vi "GT Compile.vi"(8 "error in (no error)":errorcluster caption="错误输入（无错误）", 9 "pWrongInfo":T1, 10 "pFileName":string, 11 "cardNum":i16) -> (0 "error out":errorcluster caption="错误输出", 1 "pWrongInfo out":T1, 2 "pFileName out":string, 3 "pFileName":string, 4 "function return":i16, 5 "pMessage":string)   [LabVIEW 2020, in "gts.lvlib"]
doc: "GT_API GT_Compile(short cardNum,char *pFileName,TCompileInfo *pWrongInfo);"
uses:
  gts.lvlib
  <vilib>/Utility/importsl/GetValueByPointer/datatype.ctl
  <vilib>/Utility/importsl/GetValueByPointer/GetValueByPointer.xnode
  dll/32bit/multi_card/gts.dll
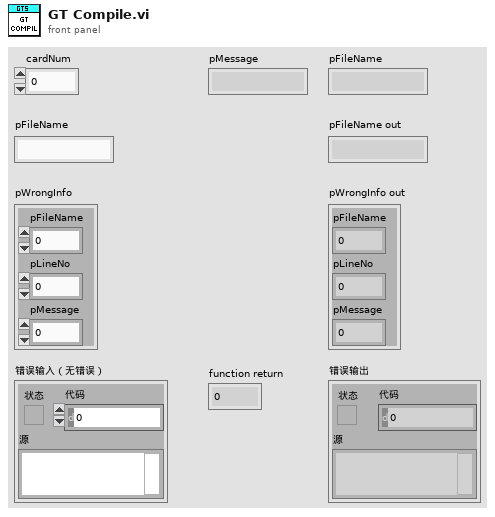
[diagram p1: front panel]
types:
  T1 = cluster{"pFileName":u32, "pLineNo":u32, "pMessage":u32}
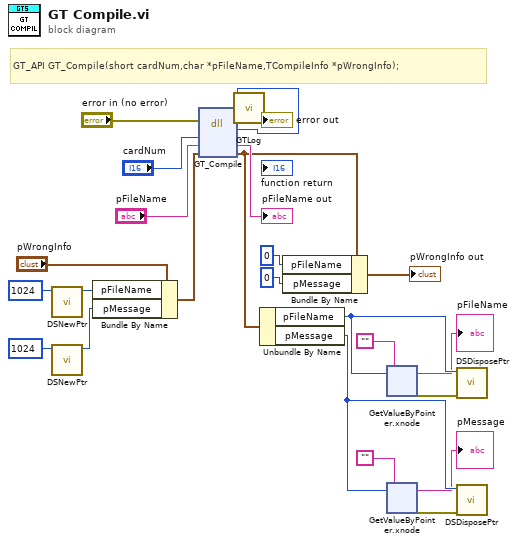
[diagram p0: block diagram]
diagram:
  # "GT_API GT_Compile(short cardNum,char *pFileName,TCompileInfo *pWrongInfo);"
  n1 = call <vilib>:"DSNewPtr.vi"("Size"=u64 1024) -> ("Pointer"=w19:u64)  [unwired: 9 in, 1 out]
  n2 = call <vilib>:"DSNewPtr.vi"("Size"=u64 1024) -> ("Pointer"=w17:u64)  [unwired: 9 in, 1 out]
  n3 = Bundle By Name(cluster="pWrongInfo", "pFileName"=w19, "pMessage"=w17) -> (w18:T1)
  n4 = dll-call lib="C:/1228/dll/32bit/multi_card/gts.dll" fn="GT_Compile"(error in="error in (no error)", "cardNum"="cardNum", "pFileName"="pFileName", "pWrongInfo"=w18) -> (error out=w3:errorcluster, w1:i16, "pFileName"=→"pFileName out":string, "pWrongInfo"=w8:T1)  [unwired: 3 in, 1 out]
  n5 = call "GTLog.vi"("error in (no error)"=w3, "Numeric"=w1) -> ("error out"=→"error out":errorcluster)  [unwired: 9 in]
  n6 = Unbundle By Name(w8) -> ("pFileName"=w15:u32, "pMessage"=w11:u32)
  n7 = Bundle By Name(cluster=w8, "pFileName"=u32 0, "pMessage"=u32 0) -> (→"pWrongInfo out":T1)
  n8 = xnode "GetValueByPointer.xnode"("Pointer"=w15, "InputType"="") -> ("Output"=→"pFileName":string, "ErrorOut"=w16:errorcluster)  [unwired: 2 in]
  n9 = xnode "GetValueByPointer.xnode"("Pointer"=w11, "InputType"="") -> ("Output"=→"pMessage":string, "ErrorOut"=w12:errorcluster)  [unwired: 2 in]
  n10 = call <vilib>:"DSDisposePtr.vi"("error in (no error)"=w16, "Pointer"=w15) -> ()  [unwired: 9 in, 1 out]
  n11 = call <vilib>:"DSDisposePtr.vi"("error in (no error)"=w12, "Pointer"=w11) -> ()  [unwired: 9 in, 1 out]
